vi "下降沿检测.vi"(8 "error in":errorcluster, 11 "input":bool) -> (0 "error out":errorcluster, 3 "output":bool)   [LabVIEW 2012, in "边沿检测.lvlib"]
uses:
  <vilib>/ptbypt/NI_PtbyPt.lvlib
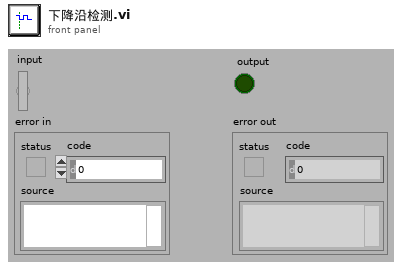
[diagram p1: front panel]
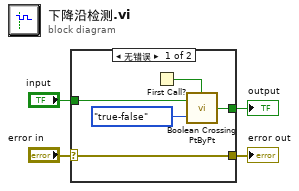
[diagram p0: block diagram]
diagram:
  n1 = case shown="无错误" "error in" {
    selector: "error in" -> [w8 w10]
    tunnel: "input" -> [w6 _]
    tunnel: [w5 _] -> w2
    tunnel: [w8 w10] -> w4
    frame No Error {
      n2 = First Call?() -> (First Call?: T/F=w7:bool)
      n3 = call <vilib>:"Boolean Crossing PtByPt.vi"("initialize"=w7, "direction"=enum16{"either", "false-true", "true-false"}."true-false", "input"=w6) -> ("crossing"=w5:bool)
    }
    frame Error {
    }
  }
  "output" <- w2
  "error out" <- w4
